vi "String Output Item.vi"(8 "error in (no error)":errorcluster, 9 "Project In":refnum<class "Project.lvclass">, 11 "Output":T2) -> (0 "error out":errorcluster)   [LabVIEW 2015, in "OutputUI.lvclass"]
uses:
  OutputUI.lvclass
  Step/STEP_OUTPUT.ctl
  Step/OUTPUT_DATA_TYPE.ctl
  OUTPUT_CHECK_TYPE.ctl
  Step/OUTPUT_VALUE_TYPE.ctl
  Project.lvclass
  SerializableObject/CONFIGURE_UI_STATE.ctl
  Editor/Editor.lvclass
  Step.lvclass
panel:
  in  "Limit Value Type":T1
  in  "Variable Name":string(combo)
  in  "Regex Setup":bool
  in  "Ignore Case":bool
  in  "String Limit":string
  in  "Check":u16(ring)
  out "Type Image":picture
  in  "Output":string
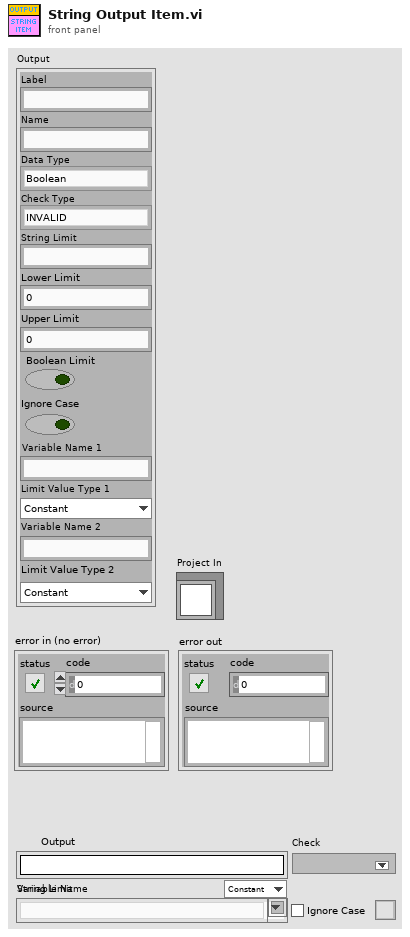
[diagram p1: front panel]
types:
  T1 = typedef "Step.lvclass/OUTPUT_VALUE_TYPE.ctl" = enum16{"Constant", "Variable"}
  T2 = typedef "Step.lvclass/STEP_OUTPUT.ctl" = cluster{"Label":string, "Name":string, "Data Type":T3, "Check Type":T4, "String Limit":string, "Lower Limit":dbl, "Upper Limit":dbl, "Boolean Limit":bool, "Ignore Case":bool, "Variable Name 1":string, "Limit Value Type 1":T1, "Variable Name 2":string, "Limit Value Type 2":T1}
  T3 = typedef "Step.lvclass/OUTPUT_DATA_TYPE.ctl" = enum16{"Boolean", "String", "Numeric", "Other"}
  T4 = typedef "Step.lvclass/OUTPUT_CHECK_TYPE.ctl" = enum16{"INVALID", "DO_NOT_CHECK", "RECORD", "VARIABLE", "EQUAL", "NOT_EQUAL", "STR_CONTAINS", "STR_START_WITH", "STR_END_WITH", "STR_REGEX_MATCH", "NUM_GT", "NUM_LT", "NUM_GE", "NUM_LE", "NUM_RANGE", "NUM_RANGE_BDY"}
  T5 = cluster{"Type Image":refnum<vi>, "Output":refnum<vi>, "Check":refnum<vi>, "String Limit":refnum<vi>, "Ignore Case":refnum<vi>, "Regex Setup":refnum<vi>, "Variable Name":refnum<vi>, "Limit Value Type":refnum<vi>}
  T6 = typedef "Editor.lvclass/CONFIGURE_UI_STATE.ctl" = enum16{"UI_LOOP", "INIT", "END", "CHANGE_PANEL"}
  T7 = typedef "LVRectTypeDef.ctl" = cluster{"Left":i16, "Top":i16, "Right":i16, "Bottom":i16}
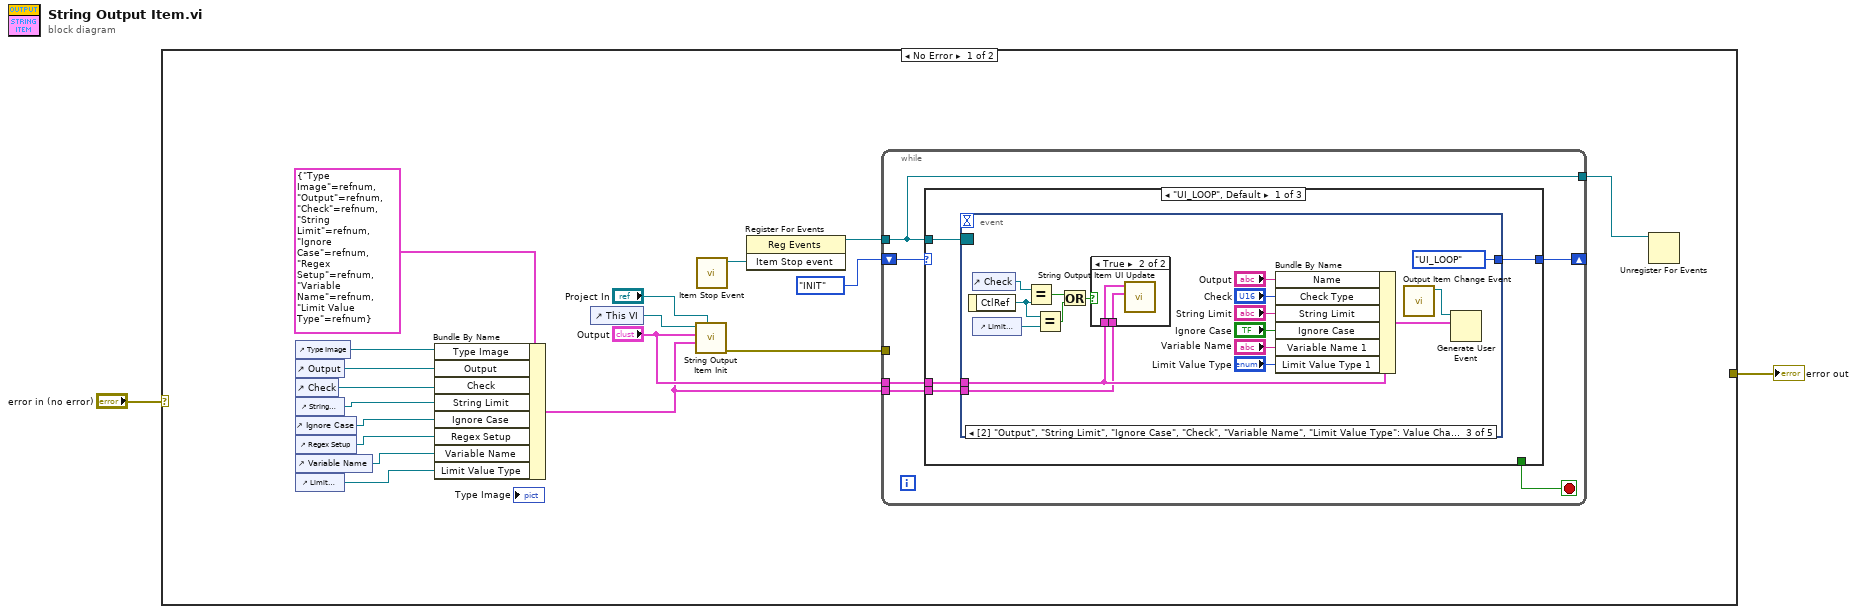
[diagram p0: block diagram]
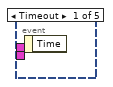
[diagram p2: hidden frame]
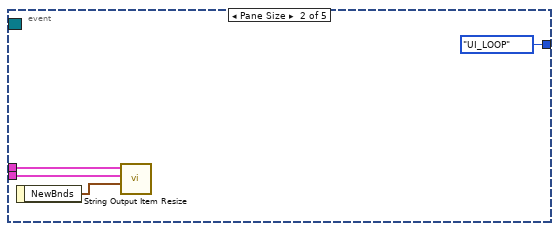
[diagram p3: hidden frame]
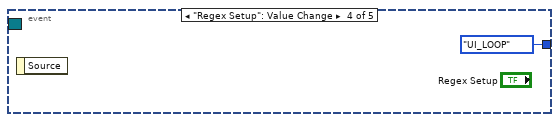
[diagram p5: hidden frame]
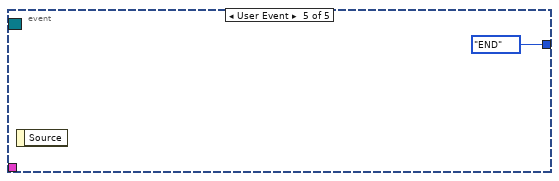
[diagram p6: hidden frame]
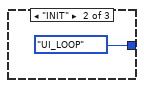
[diagram p7: hidden frame]
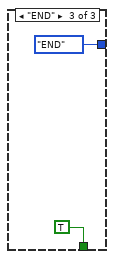
[diagram p8: hidden frame]
diagram:
  n1 = case shown="No Error" "error in (no error)" {
    selector: "error in (no error)" -> [_ w59]
    tunnel: [_ w59] -> w1
    frame No Error {
      n2 = control-ref of="Type Image"() -> (w13:refnum<vi>)
      n3 = control-ref of="Output"() -> (w9:refnum<vi>)
      n4 = control-ref of="Check"() -> (w10:refnum<vi>)
      n5 = control-ref of="String Limit"() -> (w11:refnum<vi>)
      n6 = control-ref of="Ignore Case"() -> (w6:refnum<vi>)
      n7 = control-ref of="Regex Setup"() -> (w5:refnum<vi>)
      n8 = control-ref of="Variable Name"() -> (w4:refnum<vi>)
      n9 = control-ref of="Limit Value Type"() -> (w3:refnum<vi>)
      n10 = Bundle By Name(cluster=T5 {"Type Image"=refnum, "Output"=refnum, "Check"=refnum, "String Limit"=refnum, "Ignore Case"=refnum, "Regex Setup"=refnum, "Variable Name"=refnum, "Limit Value Type"=refnum} ("UI Elements"), "Type Image"=w13, "Output"=w9, "Check"=w10, "String Limit"=w11, "Ignore Case"=w6, "Regex Setup"=w5, "Variable Name"=w4, "Limit Value Type"=w3) -> (w8:T5)
      n11 = control-ref of="This VI"() -> (w16:refnum<vi>)
      n12 = call "String Output Item Init.vi"("Project In"="Project In", "String UI Elements"=w8, "Output"="Output", "VI in"=w16) -> ("error out"=w15:errorcluster)  [unwired: 7 in]
      n13 = call "Item Stop Event.vi"() -> ("Item Stop event"=w19:refnum<user-event>)  [unwired: 11 in]
      n14 = register-events(w19) -> (reference out=w18:refnum<event-registration>)  [unwired: 2 in, 1 out]
      n15 = while {
        shift-right: [w25] -> _
        shift-left: CONFIGURE_UI_STATE."INIT" -> [w26]
        tunnel: w18 -> [w23]
        tunnel: [w23] -> w17
        tunnel: w15 -> [_]
        tunnel: "Output" -> [w22]
        tunnel: w8 -> [w21]
        stop <- w24 stop-if-true
        n16 = case shown="\"UI_LOOP\", Default" w26 {
          tunnel: [w30 CONFIGURE_UI_STATE."UI_LOOP" CONFIGURE_UI_STATE."END"] -> w25
          tunnel: [_ _ TRUE] -> w24
          tunnel: w23 -> [w29 _ _]
          tunnel: w22 -> [w28 _ _]
          tunnel: w21 -> [w27 _ _]
          frame "UI_LOOP", Default {
            n17 = event shown="[2] \"Output\", \"String Limit\", \"Ignore Case\", \"Check\", \"Variable Name\", \"Limit Value Type\": Value Change" {
              selector: w29 -> [_ _ _ _ _]
              dyn-events: _ -> [_ _ _ _ _]
              timeout: _ -> [_ _ _ _ _]
              tunnel: [_ CONFIGURE_UI_STATE."UI_LOOP" CONFIGURE_UI_STATE."UI_LOOP" CONFIGURE_UI_STATE."UI_LOOP" CONFIGURE_UI_STATE."END"] -> w30
              tunnel: w28 -> [_ w34 w44 _ _]
              tunnel: w27 -> [_ w33 w43 _ _]
              event Timeout {
                n18 = event-data() -> ()  [unwired: 1 in, 1 out]
              }
              event Pane Size {
                n19 = event-data() -> ("NewBnds"=w32:T7)  [unwired: 1 in]
                n20 = call "String Output Item Resize.vi"("NewBnds"=w32, "String UI Elements"=w33, "Output"=w34) -> ()  [unwired: 8 in, 1 out]
              }
              event "Output", "String Limit", "Ignore Case", "Check", "Variable Name": Value Change {
                n21 = event-data() -> ("CtlRef"=w39:refnum<vi>)  [unwired: 1 in]
                n22 = control-ref of="Check"() -> (w45:refnum<vi>)
                n23 = control-ref of="Limit Value Type"() -> (w38:refnum<vi>)
                n24 = Equal?(x=w45, y=w39) -> (x = y?=w36:bool)
                n25 = Equal?(x=w39, y=w38) -> (x = y?=w35:bool)
                n26 = Or(x=w36, y=w35) -> (x .or. y?=w37:bool)
                n27 = case shown="True" w37 {
                  tunnel: w44 -> [_ w53]
                  tunnel: w43 -> [_ w52]
                  frame False {
                  }
                  frame True {
                    n28 = call "String Output Item UI Update.vi"("String UI Elements"=w52, "Output"=w53) -> ()  [unwired: 9 in, 1 out]
                  }
                }
                n29 = Bundle By Name(cluster=w44, "Name"="Output", "Check Type"="Check", "String Limit"="String Limit", "Ignore Case"="Ignore Case", "Variable Name 1"="Variable Name", "Limit Value Type 1"="Limit Value Type") -> (w46:T2)
                n30 = call "Output Item Change Event.vi"() -> ("Output Value Change Event"=w47:refnum<user-event>)  [unwired: 11 in]
                n31 = Generate User Event(user event=w47, event data cluster=w46) -> ()  [unwired: 2 in, 2 out]
              }
              event "Regex Setup": Value Change {
                n32 = event-data() -> ()  [unwired: 1 in, 1 out]
              }
              event User Event {
                n33 = event-data() -> ()  [unwired: 1 in, 1 out]
              }
            }
          }
          frame "INIT" {
          }
          frame "END" {
          }
        }
      }
      n34 = Unregister For Events(event registration refnum=w17) -> ()  [unwired: 1 in, 1 out]
    }
    frame Error {
    }
  }
  "error out" <- w1
